vi "write_abc-file-test.vi"() -> ()   [LabVIEW 2012]
panel:
  out "error out":errorcluster
  in  "error in":errorcluster
  in  "File name in":path=path "C:/TEST"
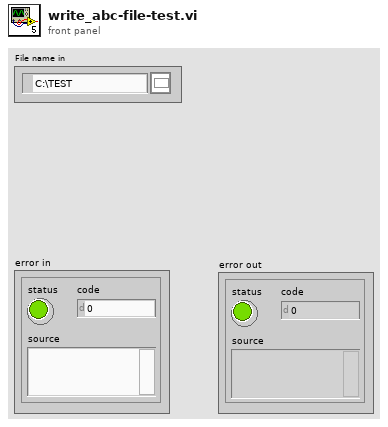
[diagram p1: front panel]
types:
  T1 = enum16{"open", "replace", "create", "open or create", "replace or create", "replace or create with confirmation"}
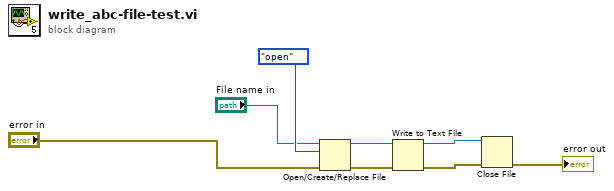
[diagram p0: block diagram]
diagram:
  n1 = Open/Create/Replace File(file path (use dialog)="File name in", error in="error in", operation (0:open)=T1."open") -> (refnum out=w4:refnum<file>, error out=w5:errorcluster)  [unwired: 4 out]
  n2 = Write to Text File(file (use dialog)=w4, error in=w5) -> (refnum out=w2:refnum<file>, error out=w3:errorcluster)  [unwired: 2 in, 1 out]
  n3 = Close File(refnum=w2, error in=w3) -> (error out=→"error out":errorcluster)  [unwired: 1 out]
